vi "Destroy Data Channels.vi"(8 "error in":errorcluster, 11 "Node in":refnum<class "AMS Chiller Template.lvclass">) -> (0 "error out":errorcluster, 3 "Node out":refnum<class "AMS Chiller Template.lvclass">)   [LabVIEW 2023, in "AMS Chiller Template.lvlib" / "AMS Chiller Template.lvclass"]
uses:
  AMS Chiller Template.lvclass
  AMS Chiller Template.lvclass/AMS Chiller Template.ctl
  C:/Program Files/National Instruments/AMS plugin/Capabilities/Capabilities/High Level Capabilities/Chiller/Chiller.lvclass
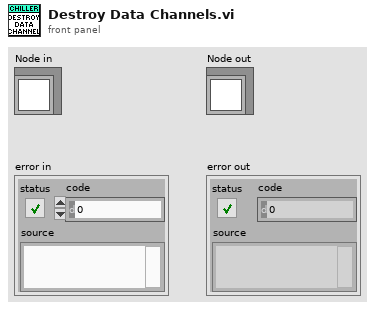
[diagram p1: front panel]
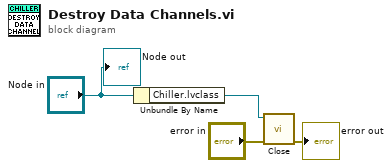
[diagram p0: block diagram]
diagram:
  n1 = Unbundle By Name("Node in") -> ("Chiller.lvclass"=w4:refnum<class "Chiller.lvclass">)
  n2 = call-dynamic "Close.vi"("error in"="error in", "Chiller in"=w4) -> ("error out"=→"error out":errorcluster)  [unwired: 8 in, 1 out]
  "Node out" <- "Node in"
